vi "UDP Buffered Rx Process.vi"(10 "Parameters":variant, 11 "Process":refnum<class "Process.lvclass">) -> ()   [LabVIEW 2016, in "UDP-Custom-Device Engine.lvlib"]
uses:
  UDP-Custom-Device Engine.lvlib
  <vilib>/NI/NIVS Inline Async API/_VS Inline Async API/Process/Process.lvclass
  <vilib>/NI/NIVS Inline Async API/_VS Inline Async API/Process/Process.lvclass/Process.ctl
  <vilib>/NI/NIVS Inline Async API/_VS Inline Async API/Process/Data Member Access/Read Data Access.vi
  <vilib>/NI/NIVS Inline Async API/_VS Inline Async API/Error Handling Process/SubVIs/Error.ConvertArray.vi
  <vilib>/NI/NIVS Inline Async API/_Data Access Engine/Data Access Engine/Data Access Engine.lvclass
  <vilib>/NI Veristand/VeriStand Data/VeriStand Data.lvlib
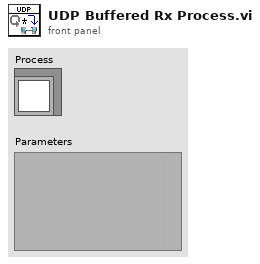
[diagram p1: front panel]
types:
  T1 = typedef "UDP-Custom-Device Engine.lvlib/Engine - Buffered Rx Loop Data.ctl" = cluster{"General Resources":T2, "Header Details":T4, "Buffer Resources":T5, "Runtime Resources":T7, "New Data Support":T10, "Buffer Option Support":T12, "Channel Resources":T16, "Debug Resources":T19}
  T2 = typedef "UDP-Custom-Device Engine.lvlib/Engine - General Resources.ctl" = cluster{"Packet Name":string, "Packet ID":i32, "Local IP Address":string, "Local Port":i32, "Multicast":bool, "Multicast IP Address":u32, "Header Info":bool[], "Byte Order":enum16{"big-endian, network order", "native, host order", "little-endian"}, "Channel Data Types":T3[], "Duplex Packets":refnum<data-value>}
  T3 = typedef "VeriStand Data.lvlib/Typedefs.Data Types.ctl" = enum16{"Boolean", "Single", "Double", "I8", "I16", "I32", "I64", "U8", "U16", "U32", "U64"}
  T4 = typedef "UDP-Custom-Device Shared.lvlib/Shared - Header Details.ctl" = cluster{"Packet Size":u16, "Protocol Revision":u8, "System Definition Version":u64, "Source Node Name":string, "Packet ID":u32, "Number of Channels":u32, "Static Header Size":u16, "Total Header Size":u16}
  T5 = typedef "UDP-Custom-Device Engine.lvlib/Engine - Buffer Resources.ctl" = cluster{"Data Buffer":u64, "Pointer Encoding":T6, "Buffer Size":u64, "Buffer Size (I32)":i32, "Raw Buffer Data":u8[], "Is Buffered":bool, "External Buffer":bool, "Prepend Header":bool, "Valid Buffer":bool}
  T6 = typedef "UDP-Custom-Device Shared.lvlib/Shared - Pointer Encoding.ctl" = enum16{"Direct Encoding", "Conversion Encoding"}
  T7 = typedef "UDP-Custom-Device Engine.lvlib/Engine - Rx Runtime Resources.ctl" = cluster{"Connection ID":refnum<k16>, "Timeout":i32, "ExecutionConfig":T8}
  T8 = typedef "UDP-Custom-Device Engine.lvlib/Engine - Execution Config.ctl" = cluster{"Loop Period":i64, "RT Loop Period":i64, "Untimed Period":u32, "Target Processor":i32, "Priority":i32, "Thread Management":T9}
  T9 = typedef "UDP-Custom-Device Shared.lvlib/Shared - Thread Management.ctl" = enum16{"Untimed (Default)", "Timed (High Priority)"}
  T10 = typedef "UDP-Custom-Device Engine.lvlib/Engine - Rx New Data Options Support.ctl" = cluster{"New Data Option":T11, "Packet Count":dbl}
  T11 = typedef "UDP-Custom-Device Shared.lvlib/Shared - New Data Options.ctl" = enum16{"Timeout Reset", "Counter"}
  T12 = typedef "UDP-Custom-Device Engine.lvlib/Engine - Buffered Rx Buffer Option Support.ctl" = cluster{"Buffer Option":T13, "Circular Buffer":T14, "Cached Buffer":T15}
  T13 = typedef "UDP-Custom-Device Shared.lvlib/Shared - Receive Buffer Options.ctl" = enum16{"Static Buffer", "Circular Buffer", "Circular Buffer + Size", "Block Cache", "Block Cache + Size"}
  T14 = typedef "UDP-Custom-Device Engine.lvlib/Engine - Buffered Rx Circular Buffer.ctl" = cluster{"Circular Offset":u64, "Size Offset":u64, "Data Offset":u64, "Null Offset":u64}
  T15 = typedef "UDP-Custom-Device Engine.lvlib/Engine - Buffered Rx Cached Buffer.ctl" = cluster{"Cache Buffer":u64, "Cache Size":u64, "Cache Size (I32)":i32, "Raw Data":u8[], "Null Buffer":u8[], "Size Offset":u64, "Data Offset":u64, "New Data Offset":u64}
  T16 = typedef "UDP-Custom-Device Engine.lvlib/Engine - Buffered Rx Channel Refs.ctl" = cluster{"New Data":T17, "Received Bytes":T17, "Port":T17, "Buffer (External)":T18, "Buffer (Local)":T17}
  T17 = typedef "Data Access Engine.lvlib/Data Access Engine.lvclass/Write.DVR.ctl" = refnum<data-value>
  T18 = typedef "Data Access Engine.lvlib/Data Access Engine.lvclass/Read.DVR.ctl" = refnum<data-value>
  T19 = typedef "UDP-Custom-Device Engine.lvlib/Engine - Debug Resources.ctl" = cluster{"Debug Mode":bool, "Debug Log File":refnum<file>, "Packet Name":string}
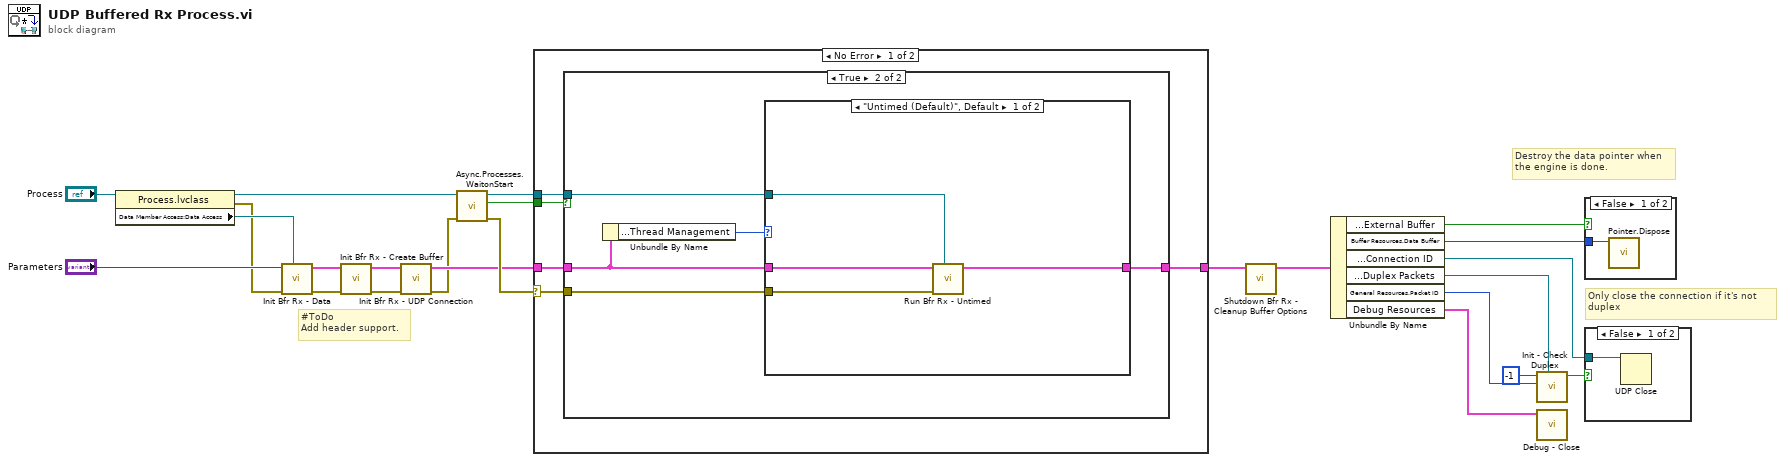
[diagram p0: block diagram]
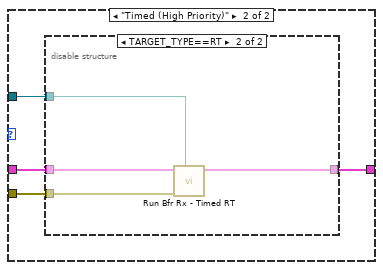
[diagram p3: hidden frame]
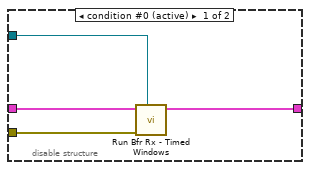
[diagram p4: hidden frame]
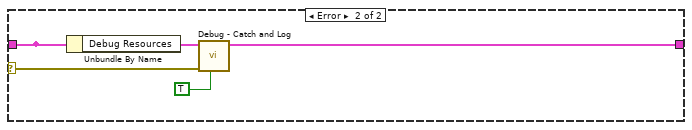
[diagram p5: hidden frame]
diagram:
  # "Only close the connection if it's not\nduplex"
  # "#ToDo\nAdd header support."
  # "Destroy the data pointer when\nthe engine is done."
  n1 = property class="Process.lvclass"(reference="Process") -> (reference out=w24:refnum<class "Process.lvclass">, error out=w17:errorcluster, "Data Member Access:Data Access"=w19:refnum<class "Data Access Engine.lvclass">)  [unwired: 1 in]
  n2 = call "Init Bfr Rx - Data.vi"("Data Access"=w19, "error in (no error)"=w17, "Parameters"="Parameters") -> ("error out"=w15:errorcluster, "Rx Loop Data"=w16:T1)  [unwired: 7 in]
  n3 = call "Init Bfr Rx - Create Buffer.vi"("error in (no error)"=w15, "Rx Loop Data in"=w16) -> ("error out"=w12:errorcluster, "Rx Loop Data out"=w14:T1)  [unwired: 8 in]
  n4 = call "Init Bfr Rx - UDP Connection.vi"("error in (no error)"=w12, "Rx Loop Data in"=w14) -> ("error out"=w11:errorcluster, "Rx Loop Data out"=w13:T1)  [unwired: 8 in]
  n5 = call <vilib>:"Async.Processes.WaitonStart.vi"("error in (no error)"=w11, "Process"=w24) -> ("error out"=w22:errorcluster, "Execute"=w20:bool, "Process out"=w21:refnum<class "Process.lvclass">)  [unwired: 7 in]
  n6 = case shown="No Error" w22 {
    selector: w22 -> [w27 w53]
    tunnel: w20 -> [w29 _]
    tunnel: w21 -> [w28 _]
    tunnel: w13 -> [w26 w52]
    tunnel: [w25 w52] -> w1
    frame No Error {
      n7 = case shown="True" w29 {
        tunnel: w27 -> [_ w34]
        tunnel: w28 -> [_ w35]
        tunnel: w26 -> [w30 w32]
        tunnel: [w30 w33] -> w25
        frame False {
        }
        frame True {
          n8 = Unbundle By Name(w32) -> ("Runtime Resources.ExecutionConfig.Thread Management"=w31:T9)
          n9 = case shown="\"Untimed (Default)\", Default" w31 {
            tunnel: w35 -> [w38 w43]
            tunnel: w34 -> [w37 w42]
            tunnel: [w36 w41] -> w33
            tunnel: w32 -> [w39 w40]
            frame "Untimed (Default)", Default {
              n10 = call "Run Bfr Rx - Untimed.vi"("Process in"=w38, "error in (no error)"=w37, "Rx Loop Data in"=w39) -> ("Rx Loop Data out"=w36:T1)  [unwired: 8 in]
            }
            frame "Timed (High Priority)" {
              n11 = disable-structure shown="TARGET_TYPE==RT" {
                disable-tunnel: w43 -> [w46 w50]
                disable-tunnel: w42 -> [w45 w49]
                disable-tunnel: w40 -> [w47 w51]
                disable-tunnel: [w44 w48] -> w41
                frame condition #0 (active) {
                  n12 = call "Run Bfr Rx - Timed Windows.vi"("Process in"=w46, "error in (no error)"=w45, "Rx Loop Data in"=w47) -> ("Rx Loop Data out"=w44:T1)  [unwired: 8 in]
                }
                frame condition #1 {
                  n13 = call "Run Bfr Rx - Timed RT.vi"("Process in"=w50, "error in (no error)"=w49, "Rx Loop Data in"=w51) -> ("Rx Loop Data out"=w48:T1)  [unwired: 8 in]
                }
              }
            }
          }
        }
      }
    }
    frame Error {
      n14 = Unbundle By Name(w52) -> ("Debug Resources"=w54:T19)
      n15 = call "Debug - Catch and Log.vi"("Clear Error?"=TRUE, "error in (no error)"=w53, "Debug Resources"=w54) -> ()  [unwired: 8 in, 1 out]
    }
  }
  n16 = call "Shutdown Bfr Rx - Cleanup Buffer Options.vi"("Rx Loop Data in"=w1) -> ("Rx Loop Data out"=w2:T1)  [unwired: 9 in, 1 out]
  n17 = Unbundle By Name(w2) -> ("Buffer Resources.External Buffer"=w9:bool, "Buffer Resources.Data Buffer"=w10:u64, "Runtime Resources.Connection ID"=w5:refnum<k16>, "General Resources.Duplex Packets"=w6:refnum<data-value>, "General Resources.Packet ID"=w4:i32, "Debug Resources"=w3:T19)
  n18 = call "Init - Check Duplex.vi"("Duplex Packets"=w6, "Receive Packet ID"=w4, "Transmit Packet ID"=-1 ("Receive Packet ID")) -> ("Is Duplex?"=w7:bool)  [unwired: 6 in, 2 out]
  n19 = call "Debug - Close.vi"("Debug Resources"=w3) -> ()  [unwired: 10 in, 1 out]
  n20 = case shown="False" w9 {
    tunnel: w10 -> [w56 _]
    frame False {
      n21 = call <vilib>:"Pointer.Dispose.vi"("pointer"=w56) -> ()  [unwired: 9 in, 2 out]
    }
    frame True {
    }
  }
  n22 = case shown="False" w7 {
    tunnel: w5 -> [w57 _]
    frame False {
      n23 = UDP Close(connection ID=w57) -> ()  [unwired: 1 in, 2 out]
    }
    frame True {
    }
  }
